vi "Read Database.vi"(8 "error in":errorcluster, 9 "delimiter":string=";", 11 "DB path array":path[](array[path])) -> (0 "error out":errorcluster, 3 "Array out":string[][](array[string]))   [LabVIEW 2014]
doc: "<B>Copyright</B>: (c) 2015 MHWirth. All rights reserved.\n\nThis subVI reads from database. It is capable of reading from xlsx, xls, and csv files. The database type is determined based on the file extension."
uses:
  <vilib>/addons/_office/excel.llb/Excel Get Data ([str]).vi
  <vilib>/Utility/file.llb/Read From Spreadsheet File (string).vi
  <vilib>/Utility/NIReport.llb/NI_report.lvclass
  <vilib>/addons/_office/NI_ReportGenerationToolkit.lvlib
  <vilib>/Utility/NIReport.llb/Excel/NI_Excel.lvclass
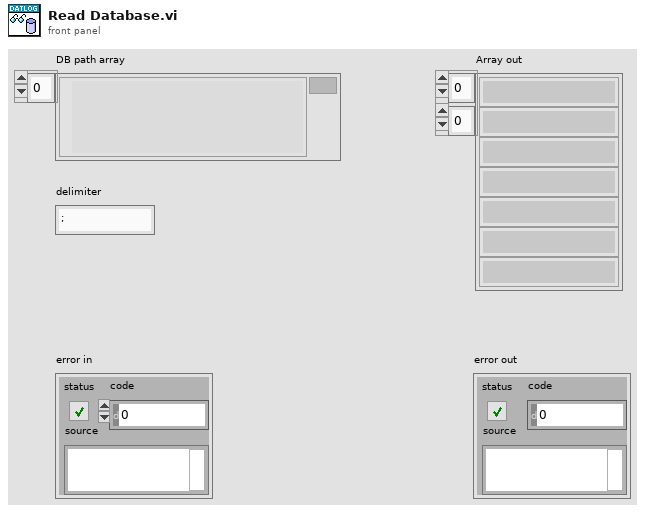
[diagram p1: front panel]
types:
  T1 = enum16{"Standard Report", "HTML", "Word", "Excel"}
  T2 = enum16{"maximized", "minimized", "normal", "no change"}
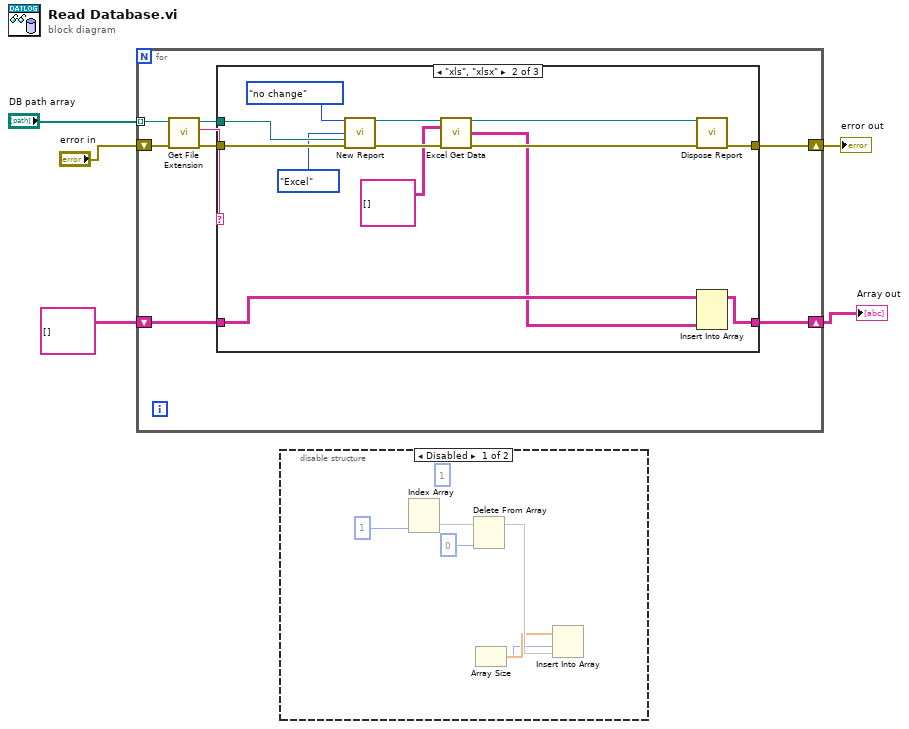
[diagram p0: block diagram]
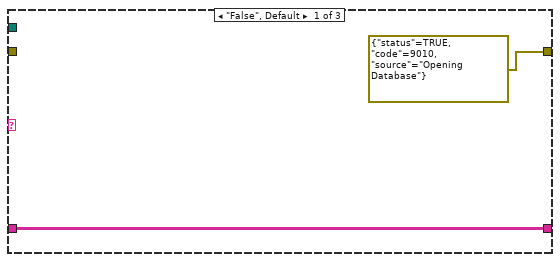
[diagram p3: hidden frame]
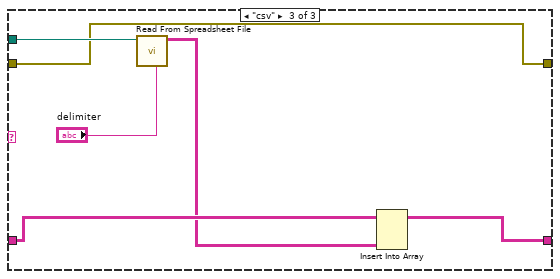
[diagram p4: hidden frame]
diagram:
  n1 = for {
    tunnel: "DB path array" -> [w13] mode=indexing
    shift-right: [w8] -> w2
    shift-left: "error in" -> [w12]
    shift-right: [w6] -> w1
    shift-left: string[][] [] -> [w7]
    n2 = call <vilib>:"Get File Extension.vi"("error in (no error)"=w12, "file"=w13) -> ("error out"=w9:errorcluster, "lowercase file extension"=w10:string, "dup file"=w11:path)  [unwired: 6 in, 1 out]
    n3 = case shown="\"xls\", \"xlsx\"" w10 {
      tunnel: w11 -> [_ w28 w34]
      tunnel: w9 -> [_ w27 w32]
      tunnel: [errorcluster {"status"=TRUE, "code"=9010, "source"="Opening Database"} ("error constant") w21 w32] -> w8
      tunnel: w7 -> [w14 w17 w31]
      tunnel: [w14 w18 w29] -> w6
      frame "False", Default {
      }
      frame "xls", "xlsx" {
        n4 = call <vilib>:"New Report.vi"("window state (normal)"=T2."no change", "report type"=T1."Excel", "template (empty)"=w28, "error in (no error)"=w27) -> ("report out"=w24:refnum<class "NI_report.lvclass">, "error out"=w23:errorcluster)  [unwired: 10 in]
        n5 = call-poly <vilib>:"Excel Get Data.vi"("report in"=w24, "data type"=string[][] [], "error in (no error)"=w23) -> ("report out"=w19:refnum<class "NI_report.lvclass">, "data"=w16:string[][], "error out"=w20:errorcluster)  [unwired: 10 in]
        n6 = call-dynamic "Dispose Report.vi"("report in"=w19, "error in (no error)"=w20) -> ("error out"=w21:errorcluster)  [unwired: 13 in]
        n7 = Insert Into Array(array=w17, new element=w16) -> (w18:string[][])  [unwired: 2 in]
      }
      frame "csv" {
        n8 = call-poly <vilib>:"Read From Spreadsheet File.vi"("delimiter (\\t)"="delimiter", "file path (dialog if empty)"=w34) -> ("all rows"=w30:string[][])  [unwired: 5 in, 4 out]
        n9 = Insert Into Array(array=w31, new element=w30) -> (w29:string[][])  [unwired: 2 in]
      }
    }
  }
  "Array out" <- w1
  "error out" <- w2
  n10 = disable-structure shown="Disabled" {
    frame Disabled {
      (unwired) 1 ("length")
      n11 = Index Array(index (col)=1 ("disabled index (col)")) -> (element=w38)  [unwired: 2 in]
      n12 = Delete From Array(array=w38, index=0) -> (length=w39:i32, array with subset deleted=w41)  [unwired: 1 out]
      n13 = Array Size() -> (array=w37:dbl[], size(s)=w36:i32)
      n14 = Insert Into Array(array=w37, index=w36, new element=w41) -> ()  [unwired: 1 out]
    }
    frame Enabled {
    }
  }
